vi "LVClass_CameraSet Get Parameter Name.vi"(0 "CameraSet.lvclass":refnum<class "CameraSet.lvclass">, 5 "index":u32, 11 "error in (no error)":errorcluster) -> (4 "CameraSet.lvclass":refnum<class "CameraSet.lvclass">, 6 "parameter_name":string, 15 "error out":errorcluster)   [LabVIEW 2020, in "CameraSet.lvclass"]
doc: "Camera parameter name getter given its position in the parameters list.\n\n<B>camera_setIn</B> : CameraSet object.\n<B>camera_setOut</B> : CameraSet object.\n<B>index</B> : Parameter index.\n<B>parameter_name</B> : Parameter name."
uses:
  CameraSet.lvclass
  CameraSet.lvclass/CameraSet.ctl
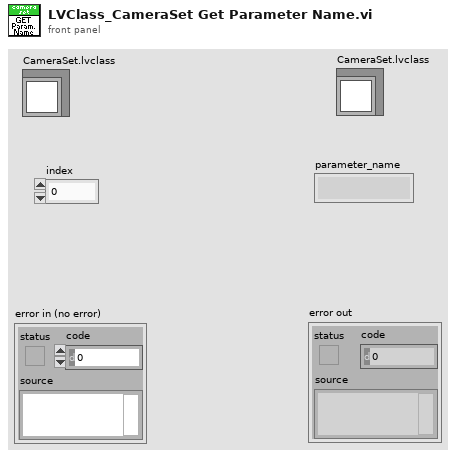
[diagram p1: front panel]
types:
  T1 = typedef "ClassID.ctl" = i64
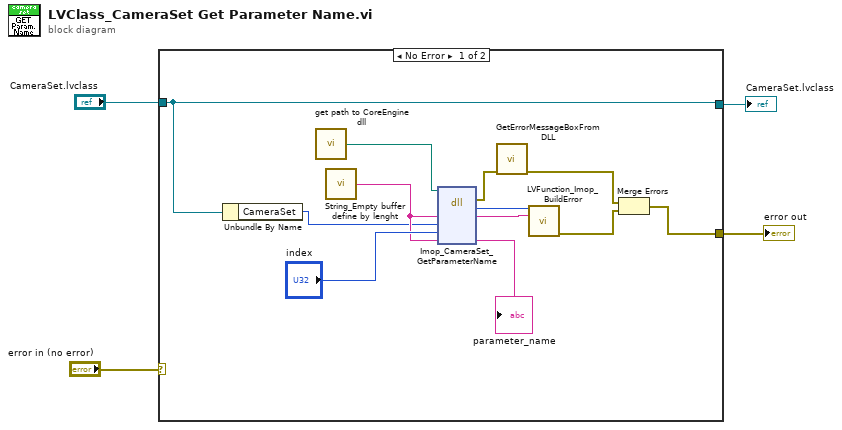
[diagram p0: block diagram]
diagram:
  n1 = case shown="No Error" "error in (no error)" {
    selector: "error in (no error)" -> [_ w17]
    tunnel: "CameraSet.lvclass" -> [w9 w18]
    tunnel: [w9 w18] -> w2
    tunnel: [w5 w17] -> w1
    frame No Error {
      n2 = Unbundle By Name(w9) -> ("CameraSet"=w8:T1)
      n3 = call "get path to CoreEngine dll.vi"() -> ("path to wavekit library"=w11:path)  [unwired: 14 in, 1 out]
      n4 = call "String_Empty buffer define by lenght.vi"() -> ("Empty buffer"=w12:string)  [unwired: 1 in]
      n5 = dll-call lib="D:/2_trunk/temp_core_engine/DLLs/ImopEngine4_vc100.dll" fn="Imop_CameraSet_GetParameterName"(path in=w11, "message"=w12, "objet"=w8, "index"="index", "parameter_name"=w12) -> (error out=w10:errorcluster, "return type"=w16:i32, "message"=w15:string, "parameter_name"=→"parameter_name":string)  [unwired: 4 in, 1 out]
      n6 = call "GetErrorMessageBoxFromDLL.vi"("error IN"=w10) -> ("error OUT"=w7:errorcluster)  [unwired: 10 in]
      n7 = call "LVFunction_Imop_BuildError.vi"("code"=w16, "String to Prepend to source (\"\")"=w15) -> ("error out"=w6:errorcluster)  [unwired: 13 in]
      n8 = Merge Errors(w7, w6) -> (w5:errorcluster)
    }
    frame Error {
    }
  }
  "CameraSet.lvclass" <- w2
  "error out" <- w1
